vi "Write Voltage Setting.vi"(0 "VISA resource name":refnum<visa-resource-name>, 1 "Enable Voltage Inversion (T: Enabled)":bool=TRUE, 7 "Voltage Setting (100.00)":dbl=100.0 format="%.2f", 11 "error in (no error)":errorcluster) -> (4 "VISA resource name out":refnum<visa-resource-name>, 15 "error out":errorcluster)   [LabVIEW 2020, in "Stanford Research PS300 Series.lvlib"]
doc: "This VI sets the output value and causes the instrument to output voltage. \n\nIf having problems setting output voltage, voltage limit, or current limit, try negating your voltage or current value."
uses:
  Stanford Research PS300 Series.lvlib
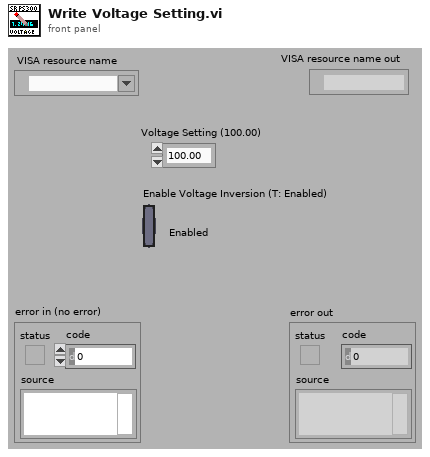
[diagram p1: front panel]
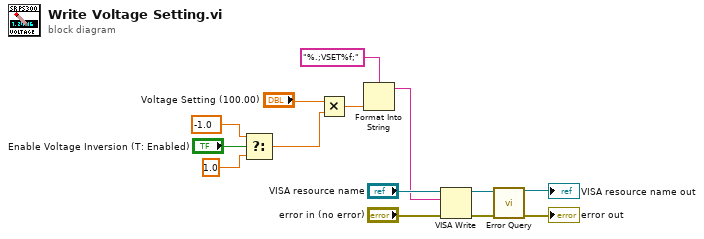
[diagram p0: block diagram]
diagram:
  n1 = Select(t=-1.0 ("y"), s="Enable Voltage Inversion (T: Enabled)", f=1.0) -> (s? t:f=w5:dbl)
  n2 = Multiply(x="Voltage Setting (100.00)", y=w5) -> (x*y=w9:dbl)
  n3 = Format Into String(format string="%.;VSET%f;", w9) -> (resulting string=w12:string)  [unwired: 2 in, 1 out]
  n4 = VISA Write(VISA resource name="VISA resource name", write buffer=w12, error in (no error)="error in (no error)") -> (VISA resource name out=w4:refnum<visa-resource-name>, error out=w3:errorcluster)  [unwired: 1 out]
  n5 = call "Error Query.vi"("VISA resource name"=w4, "error in (no error)"=w3) -> ("VISA resource name out"=→"VISA resource name out":refnum<visa-resource-name>, "error out"=→"error out":errorcluster)  [unwired: 10 in, 2 out]
